vi "Execute.vi"(8 "error in (no error)":errorcluster, 11 "SimpleAdder in":refnum<class "SimpleAdder.lvclass">) -> (0 "error out":errorcluster, 3 "SimpleAdder out":refnum<class "SimpleAdder.lvclass">)   [LabVIEW 2012]
uses:
  SimpleAdder.lvclass
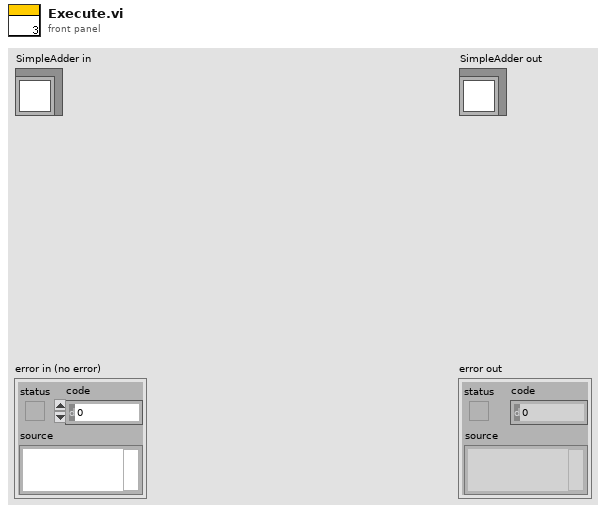
[diagram p1: front panel]
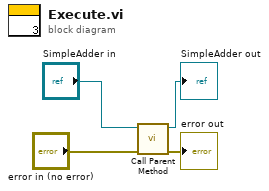
[diagram p0: block diagram]
diagram:
  n1 = call-parent "Call Parent Method"("error in (no error)"="error in (no error)", "ParentClass in"="SimpleAdder in") -> ("error out"=→"error out":errorcluster, "ParentClass out"=→"SimpleAdder out":refnum<class "SimpleAdder.lvclass">)  [unwired: 8 in]
